vi "PID EGU to %.vi"   [LabVIEW 2017, in "NI_PID_pid.lvlib"]
doc: "Converts engineering units input to percent of range output based on the minimum and maximum range settings. You can use this polymorphic VI to operate on a single input value or on an array of input values. The DBL instance can be used to implement a single control loop, whereas the DBL Array instance can be used to implement parallel multi-loop control."
uses:
  <vilib>/addons/control/pid/NI_PID_pid.lvlib
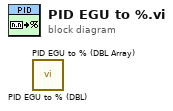
[diagram p0: block diagram]
diagram:
  n1 = call <vilib>:"PID EGU to % (DBL).vi"() -> ()  [unwired: 3 in, 1 out]
  n2 = call <vilib>:"PID EGU to % (DBL Array).vi"() -> ()  [unwired: 3 in, 1 out]
